vi "ConnectToLabJack.vi"(8 "Error In":errorcluster, 11 "Serial Number":string) -> (0 "Error Out":errorcluster, 3 "LabJack out":refnum<k24>)   [LabVIEW 2018, in "ThorlabsLabJack.lvlib" / "ThorlabsLabJack.lvclass"]
uses:
  ThorlabsLabJack.lvclass
  C:/Projects/LabVIEW/In-Progress/Chetan Malpure/Axis/Thorlabs LabJack/Drivers/Thorlabs.MotionControl.IntegratedStepperMotorsCLI.dll
  Drivers/Thorlabs.MotionControl.IntegratedStepperMotorsCLI.dll
  d21497f4-289c-4137-8a37-2b036c35e6b7.vi
  45f68063-f2cc-47e6-b36d-63514a27fa94.vi
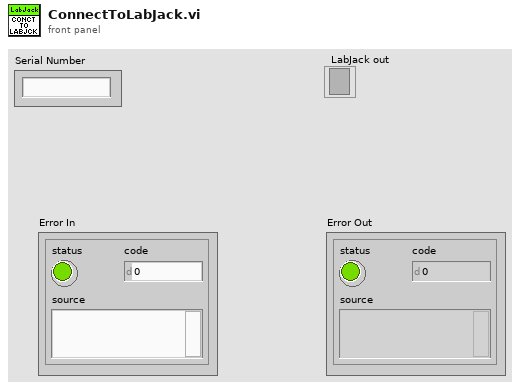
[diagram p1: front panel]
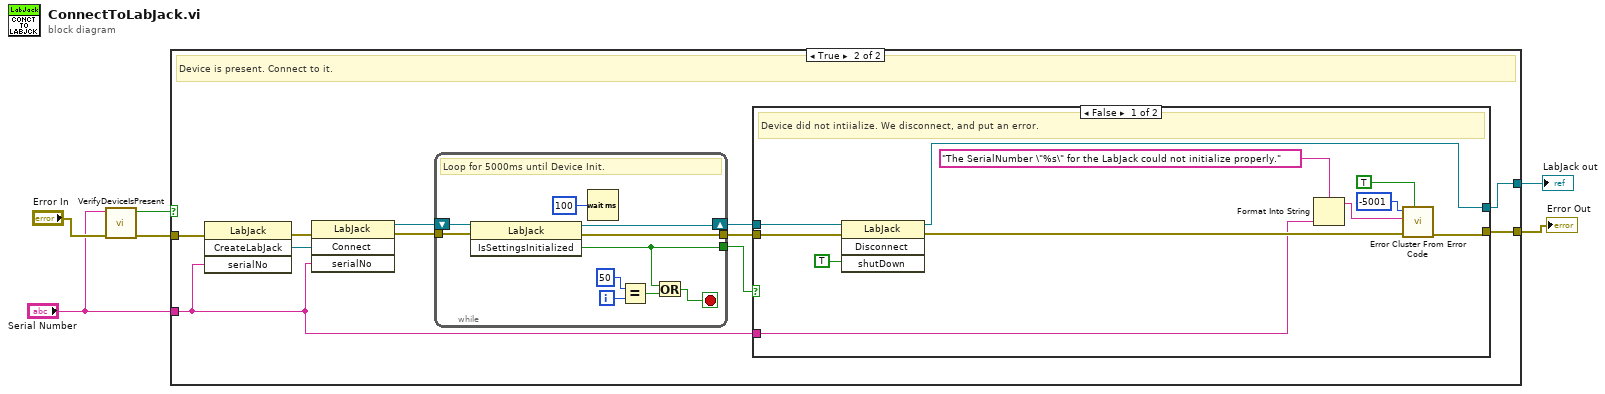
[diagram p0: block diagram]
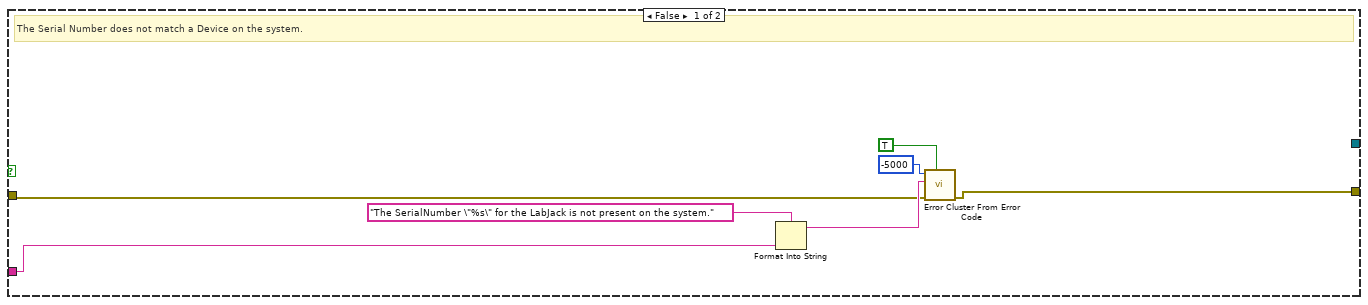
[diagram p2: hidden frame]
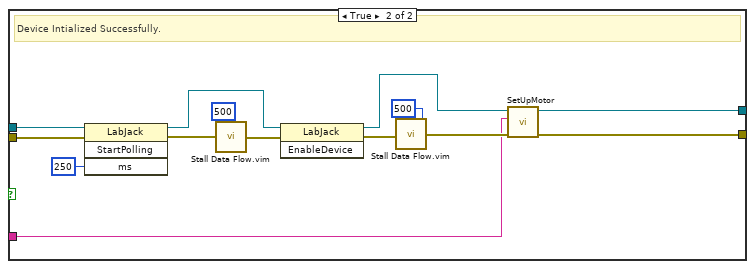
[diagram p3: hidden frame]
diagram:
  n1 = call "VerifyDeviceIsPresent.vi"("Error In"="Error In", "Serial Number in"="Serial Number") -> ("Error Out"=w5:errorcluster, "Present?"=w6:bool)  [unwired: 8 in]
  n2 = case shown="True" w6 {
    tunnel: w5 -> [w9 w23]
    tunnel: "Serial Number" -> [w8 w17]
    tunnel: [w7 w24] -> w4
    tunnel: [_ w14] -> w2
    frame False {
      # "The Serial Number does not match a Device on the system."
      n3 = Format Into String(format string="The SerialNumber \"%s\" for the LabJack is not present on the system." ("error message (\"\")"), w8) -> (resulting string=w12:string)  [unwired: 2 in, 1 out]
      n4 = call <vilib>:"Error Cluster From Error Code.vi"("show call chain? (False)"=TRUE, "error in (no error)"=w9, "error message (\"\")"=w12, "error code (0)"=-5000) -> ("error out"=w7:errorcluster)  [unwired: 5 in]
    }
    frame True {
      # "Device is present. Connect to it."
      n5 = invoke class="LabJack" method="CreateLabJack"(error in=w23, "serialNo"=w17) -> (error out=w22:errorcluster, "CreateLabJack"=w21:refnum<k24>)  [unwired: 2 in, 2 out]
      n6 = invoke class="LabJack" method="Connect"(reference=w21, error in=w22, "serialNo"=w17) -> (reference out=w19:refnum<k24>, error out=w20:errorcluster)  [unwired: 1 in, 2 out]
      n7 = while {
        tunnel: w20 -> [w53]
        shift-right: [w52] -> w16
        shift-left: w19 -> [w54]
        tunnel: [w51] -> w15
        tunnel: [w50] -> w18
        i -> [w56]
        stop <- w57 stop-if-true
        # "Loop for 5000ms until Device Init."
        n8 = invoke class="LabJack" method="IsSettingsInitialized"(reference=w54, error in=w53) -> (reference out=w52:refnum<k24>, error out=w51:errorcluster, "IsSettingsInitialized"=w50:bool)  [unwired: 1 in]
        n9 = Wait (ms)(milliseconds to wait=u32 100) -> ()  [unwired: 1 out]
        n10 = Equal?(x=50, y=w56) -> (x = y?=w59:bool)
        n11 = Or(x=w50, y=w59) -> (x .or. y?=w57:bool)
      }
      n12 = case shown="False" w18 {
        tunnel: [w31 w49] -> w24
        tunnel: w17 -> [w25 w37]
        tunnel: w16 -> [w29 w48]
        tunnel: w15 -> [w30 w47]
        tunnel: [w26 w36] -> w14
        frame False {
          # "Device did not intiialize. We disconnect, and put an error."
          n13 = invoke class="LabJack" method="Disconnect"(reference=w29, error in=w30, "shutDown"=TRUE) -> (reference out=w26:refnum<k24>, error out=w27:errorcluster)  [unwired: 1 in, 2 out]
          n14 = Format Into String(format string="The SerialNumber \"%s\" for the LabJack could not initialize properly." ("error message (\"\")"), w25) -> (resulting string=w34:string)  [unwired: 2 in, 1 out]
          n15 = call <vilib>:"Error Cluster From Error Code.vi"("show call chain? (False)"=TRUE, "error in (no error)"=w27, "error message (\"\")"=w34, "error code (0)"=-5001) -> ("error out"=w31:errorcluster)  [unwired: 5 in]
        }
        frame True {
          # "Device Intialized Successfully."
          n16 = invoke class="LabJack" method="StartPolling"(reference=w48, error in=w47, "ms"=250) -> (reference out=w42:refnum<k24>, error out=w44:errorcluster)  [unwired: 1 in, 2 out]
          n17 = call "Stall Data Flow.vim"("value in"=w44, "milliseconds to wait"=u32 500) -> ("value out"=w43:errorcluster)  [unwired: 1 out]
          n18 = invoke class="LabJack" method="EnableDevice"(reference=w42, error in=w43) -> (reference out=w40:refnum<k24>, error out=w41:errorcluster)  [unwired: 1 in, 1 out]
          n19 = call "Stall Data Flow.vim"("value in"=w41, "milliseconds to wait"=u32 500) -> ("value out"=w38:errorcluster)  [unwired: 1 out]
          n20 = call "SetUpMotor.vi"("Error In"=w38, "Serial Number"=w37, "LabJack in"=w40) -> ("Error Out"=w49:errorcluster, "LabJack out"=w36:refnum<k24>)  [unwired: 7 in]
        }
      }
    }
  }
  "Error Out" <- w4
  "LabJack out" <- w2
